vi "DEV Get Dll Build Time.vi"(11 "pDateTime":string) -> (2 "function return":u8, 3 "pDateTime out":string)   [LabVIEW 2010, in "usb_device.lvlib"]
doc: "unsigned char WINAPI DEV_GetDllBuildTime(char* pDateTime);"
uses:
  usb_device.lvlib
  USB2XXX/trunk/USB2XXX/USB2XXX/vs2019/Release/USB2XXX.dll
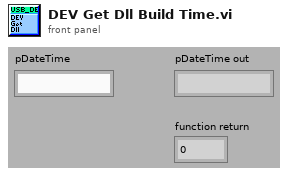
[diagram p1: front panel]
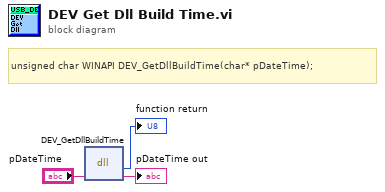
[diagram p0: block diagram]
diagram:
  # "unsigned char WINAPI DEV_GetDllBuildTime(char* pDateTime);"
  n1 = dll-call lib="E:/Projects/USB2XXX/trunk/USB2XXX/USB2XXX/vs2019/Release/USB2XXX.*" fn="DEV_GetDllBuildTime"("pDateTime"="pDateTime") -> (→"function return":u8, "pDateTime"=→"pDateTime out":string)  [unwired: 3 in, 2 out]
